vi "Query Digital State.vi"(8 "error in (no error)":errorcluster, 10 "Line Number (1: line1)":i32(ring)=1 items=["line1"=1, "line2"=2, "line3"=3, "line4"=4, "line5"=5, "line6"=6], 11 "VISA resource name":refnum<visa-resource-name>) -> (0 "error out":errorcluster, 2 "State (T: On)":bool=TRUE, 3 "VISA resource name out":refnum<visa-resource-name>)   [LabVIEW 2016, in "Keithley DMM6500 DAQ6500 Series.lvlib"]
doc: "Queries a digital I/O line high or low when the line is set for digital control and returns the state on the digital I/O lines"
uses:
  Keithley DMM6500 DAQ6500 Series.lvlib
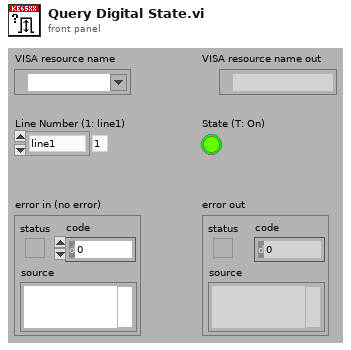
[diagram p1: front panel]
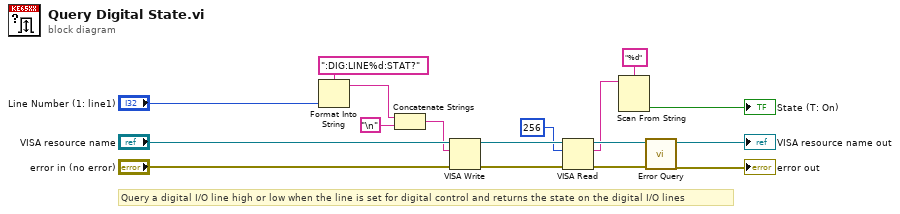
[diagram p0: block diagram]
diagram:
  # "Query a digital I/O line high or low when the line is set for digital control and returns the state on the digital I/O lines"
  n1 = Format Into String(format string=":DIG:LINE%d:STAT?", "Line Number (1: line1)") -> (resulting string=w10:string)  [unwired: 2 in, 1 out]
  n2 = Concatenate Strings(w10, "\n") -> (w11:string)
  n3 = VISA Write(VISA resource name="VISA resource name", write buffer=w11, error in (no error)="error in (no error)") -> (VISA resource name out=w6:refnum<visa-resource-name>, error out=w5:errorcluster)  [unwired: 1 out]
  n4 = VISA Read(VISA resource name=w6, byte count=u32 256, error in (no error)=w5) -> (VISA resource name out=w8:refnum<visa-resource-name>, read buffer=w3:string, error out=w7:errorcluster)  [unwired: 1 out]
  n5 = Scan From String(format string="%d", input string=w3) -> (output 1=→"State (T: On)":bool)  [unwired: 3 in, 3 out]
  n6 = call "Error Query.vi"("error in (no error)"=w7, "VISA resource name"=w8) -> ("error out"=→"error out":errorcluster, "VISA resource name out"=→"VISA resource name out":refnum<visa-resource-name>)  [unwired: 6 in, 2 out]
